vi "Configure Channels.vi"(8 "error in (no error)":errorcluster, 11 "DIO DAQmx PWM CFG in":refnum<class "DIO DAQmx PWM CFG.lvclass">) -> (0 "error out":errorcluster, 3 "DIO DAQmx PWM CFG out":refnum<class "DIO DAQmx PWM CFG.lvclass">)   [LabVIEW 2023, in "DIO DAQmx PWM CFG.lvclass"]
uses:
  DIO DAQmx PWM CFG.lvclass
  DAQmx/DAQmx Base CFG.lvclass/DAQmx Base CFG.ctl
  16d5a8d0-639b-4540-9b42-4873bb7ae69b.vi
  <vilib>/JDP Science/JSONtext/Find Item.vi
  <vilib>/JDP Science/JSONtext/Next JSON Value.vi
  <vilib>/JDP Science/JSONtext/String Subset.vi
  <vilib>/JDP Science/JSONtext/Parsing/Advance past next JSON Value (inlined COPY).vi
  <vilib>/JDP Science/JSONtext/Parsing/Advance past whitespace.vi
  <vilib>/JDP Science/JSONtext/Parsing/Advance past String.vi
  <vilib>/JDP Science/JSONtext/Parsing/Advance past Number.vi
  <vilib>/JDP Science/JSONtext/Parsing/Advance past Line Ending.vi
  <vilib>/JDP Science/JSONtext/Parsing/Parse Full Path or Item Name.vi
  <vilib>/JDP Science/JSONtext/Parsing/Advance past Array.vi
  <vilib>/JDP Science/JSONtext/Parsing/Advance past Object.vi
  <vilib>/JDP Science/JSONtext/support/Error Cluster From Code.vi
  <vilib>/JDP Science/JSONtext/Offset/Find Item Locations by Path.vi
  <vilib>/JDP Science/JSONtext/JSON text to Variant.vi
  <vilib>/Utility/error.llb/Error Cluster From Error Code.vi
  <vilib>/JDP Science/JSONtext/LVClass Serializer/JSONtext LVClass Serializer.lvclass
  <vilib>/ErrorRing/Error Ring.xnode
  DIO DAQmx PWM CFG.lvclass/DIO DAQmx PWM CFG.ctl
  <vilib>/DAQmx/create/channels.llb/DAQmx Create Channel (CO-Pulse Generation-Frequency).vi
  Configuration JSON Base/CFG JSON Base.lvclass
  DAQmx/DAQmx Base CFG.lvclass
  E:/git/HAL/HAL GOOP4/DIO/DIO DAQmx Base CFG/DIO DAQmx Base CFG.lvclass
  E:/git/HAL/HAL GOOP4/DAQmx/DAQmx Base CFG.lvclass
  E:/git/HAL/HAL GOOP4/Configuration JSON Base/CFG JSON Base.lvclass
  E:/git/HAL/HAL GOOP4/Interfaces/IConfigure/IConfigure.lvclass
  E:/git/HAL/HAL GOOP4/DIO/DIO DAQmx PWM CFG/DIO DAQmx PWM CFG.lvclass
panel:
  out "Idle State":i32(ring)=10214 items=["High"=10192, "Low"=10214]
  out "Units":i32(ring)=10373 items=["Hz"=10373]
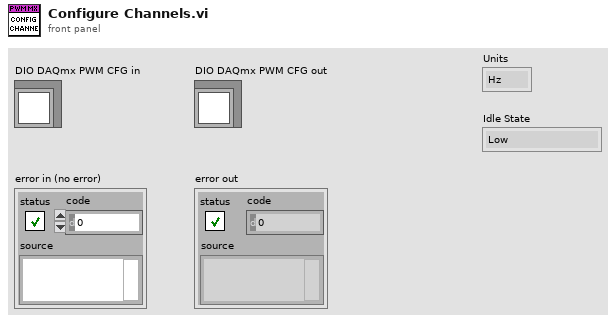
[diagram p1: front panel]
types:
  T1 = cluster{"Name":string, "Enabled":bool, "Duty Cycle":dbl, "Frequency":dbl, "Units":string, "Idle State":string, "Initial Delay":dbl}[]
  T2 = typedef "LVStringsAndValuesArrayTypeDef_I32.ctl" = cluster{"String":string, "Value":i32}[]
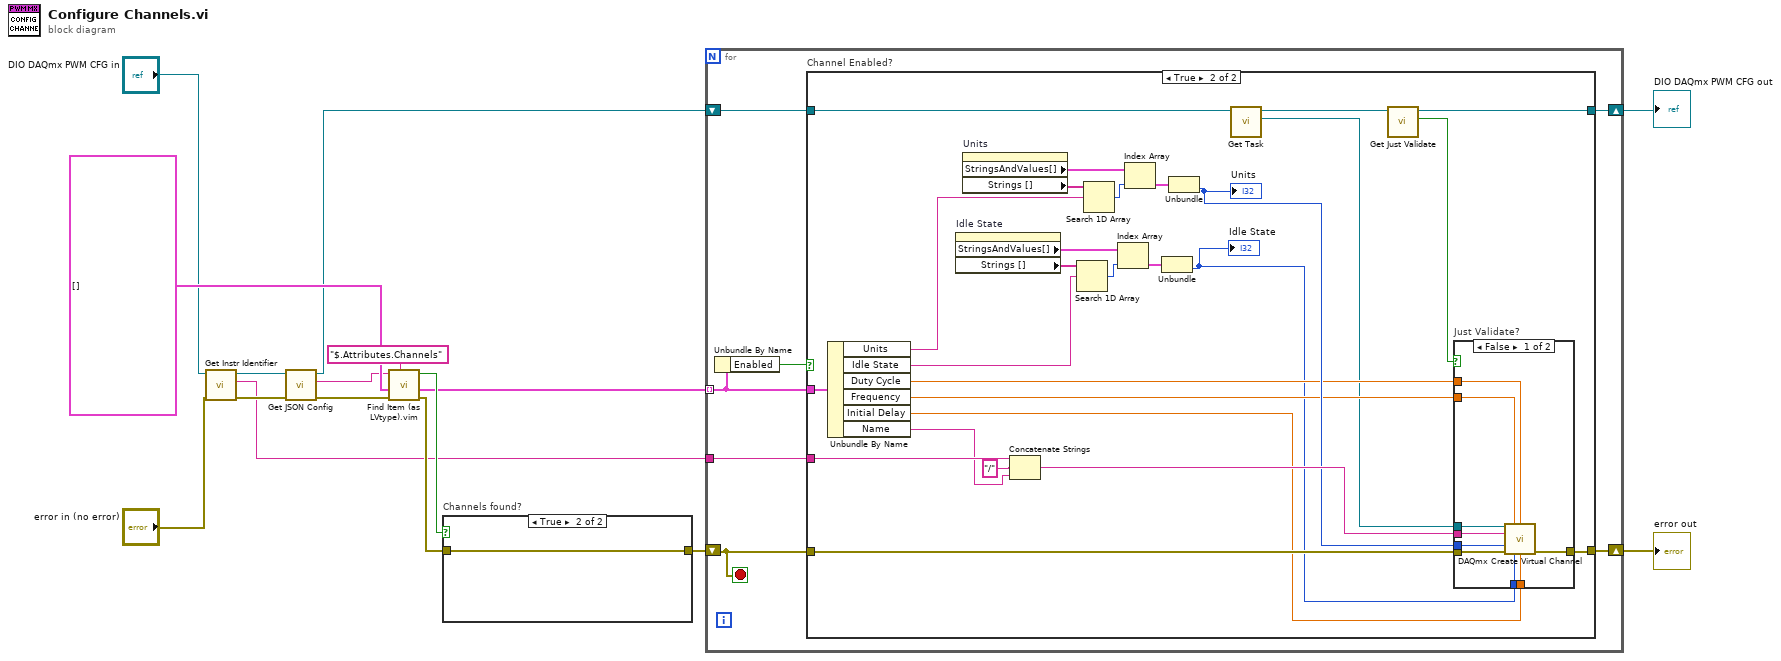
[diagram p0: block diagram]
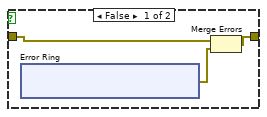
[diagram p4: hidden frame]
diagram:
  n1 = call-dynamic "Get Instr Identifier.vi"("error in (no error)"="error in (no error)", "Configuration Base in"="DIO DAQmx PWM CFG in") -> ("error out"=w8:errorcluster, "Instr Identifier"=w6:string, "Configuration Base out"=w7:refnum<class "DIO DAQmx PWM CFG.lvclass">)  [unwired: 7 in]
  n2 = call "Get JSON Config.vi"("error in (no error)"=w8, "CFG Base in"=w7) -> ("error out"=w15:errorcluster, "<JSON>Config>"=w9:string, "CFG Base out"=w2:refnum<class "DIO DAQmx PWM CFG.lvclass">)  [unwired: 7 in]
  n3 = call "Find Item (as LVtype).vim"("$Path or Item Name"="$.Attributes.Channels", "error in (no error)"=w15, "Data Type and Default Value"=T1 [], "JSON"=w9) -> ("error out"=w13:errorcluster, "Data"=w11:T1, "Found"=w14:bool)  [unwired: 4 in, 1 out]
  n4 = case "Channels found?" shown="True" w14 {
    tunnel: w13 -> [w19 w25]
    tunnel: [w17 w25] -> w12
    frame False {
      n5 = xnode "Error Ring"() -> ("error out"=w18:errorcluster)
      n6 = Merge Errors(w19, w18) -> (w17:errorcluster)
    }
    frame True {
    }
  }
  n7 = for {
    tunnel: w11 -> [w29] mode=indexing
    shift-right: [w32] -> w3
    shift-left: w12 -> [w31]
    tunnel: w6 -> [w30]
    shift-right: [w27] -> w1
    shift-left: w2 -> [w26]
    stop <- w31 stop-if-true
    n8 = Unbundle By Name(w29) -> ("Enabled"=w28:bool)
    n9 = case "Channel Enabled?" shown="True" w28 {
      tunnel: [w34 w39] -> w32
      tunnel: w31 -> [w34 w54]
      tunnel: w30 -> [_ w52]
      tunnel: w29 -> [_ w50]
      tunnel: [w33 w36] -> w27
      tunnel: w26 -> [w33 w37]
      frame False {
      }
      frame True {
        n10 = Unbundle By Name(w50) -> ("Units"=w55:string, "Idle State"=w45:string, "Duty Cycle"=w44:dbl, "Frequency"=w43:dbl, "Initial Delay"=w41:dbl, "Name"=w51:string)
        n11 = property on="Idle State" class="Ring (strict)"() -> ("StringsAndValues[]"=w61:T2, "Strings []"=w47:string[])  [unwired: 2 in, 2 out]
        n12 = property on="Units" class="Ring (strict)"() -> ("StringsAndValues[]"=w57:T2, "Strings []"=w56:string[])  [unwired: 2 in, 2 out]
        n13 = Concatenate Strings(w52, "/" ("string"), w51) -> (w49:string)
        n14 = Search 1D Array(1D array=w47, element=w45) -> (index of element=w46:i32)  [unwired: 1 in]
        n15 = Search 1D Array(1D array=w56, element=w55) -> (index of element=w58:i32)  [unwired: 1 in]
        n16 = Index Array(array=w61, index=w46) -> (element=w60:cluster{"String":string, "Value":i32})
        n17 = Index Array(array=w57, index=w58) -> (element=w59:cluster{"String":string, "Value":i32})
        n18 = Unbundle(w60) -> ("Value"=w42:i32)  [unwired: 1 out]
        "Idle State" <- w42
        n19 = Unbundle(w59) -> ("Value"=w48:i32)  [unwired: 1 out]
        "Units" <- w48
        n20 = call "Get Task.vi"("DAQmx Base CFG in"=w37) -> ("Task"=w40:refnum<k21>, "DAQmx Base CFG out"=w38:refnum<class "DIO DAQmx PWM CFG.lvclass">)  [unwired: 8 in, 1 out]
        n21 = call "Get Just Validate.vi"("CFG JSON Base in"=w38) -> ("Just Validate"=w35:bool, "CFG JSON Base out"=w36:refnum<class "DIO DAQmx PWM CFG.lvclass">)  [unwired: 8 in, 1 out]
        n22 = case "Just Validate?" shown="False" w35 {
          tunnel: w54 -> [w70 w71]
          tunnel: w49 -> [w69 _]
          tunnel: w48 -> [w68 _]
          tunnel: w44 -> [w67 _]
          tunnel: w43 -> [w66 _]
          tunnel: w42 -> [w65 _]
          tunnel: w41 -> [w64 _]
          tunnel: w40 -> [w63 _]
          tunnel: [w62 w71] -> w39
          frame False {
            n23 = call-poly <vilib>:"DAQmx Create Virtual Channel.vi"("task in"=w63, "frequency"=w66, "duty cycle"=w67, "counter"=w69, "units"=w68, "error in"=w70, "idle state"=w65, "initial delay"=w64) -> ("error out"=w62:errorcluster)  [unwired: 6 in, 1 out]
          }
          frame True {
          }
        }
      }
    }
  }
  "error out" <- w3
  "DIO DAQmx PWM CFG out" <- w1
